vi "CollisionAvoidance.vi"(8 "error in":errorcluster) -> (0 "error out":errorcluster)   [LabVIEW 2009, in "Main.lvlib"]
doc: "Collision Avoidance algorithm. Check if there is an obstacle in front and aborts position control if any."
uses:
  Main.lvlib
  Drive.lvlib
  MainVariables.lvlib
  ImageProject/Camera.lvlib
  NetworkVarTarget.lvlib
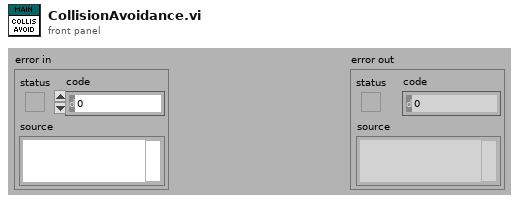
[diagram p1: front panel]
types:
  T1 = typedef "IMAQ Image.ctl" = refnum<image>
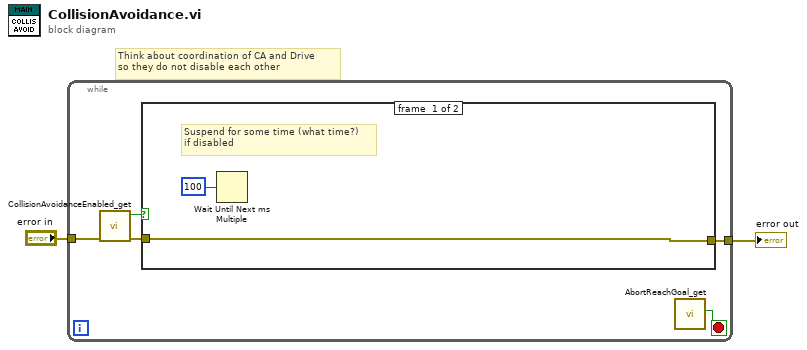
[diagram p0: block diagram]
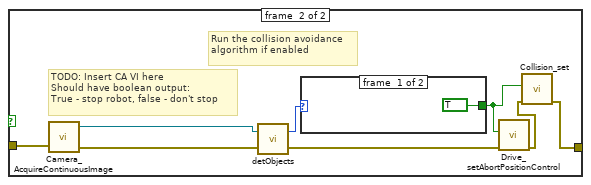
[diagram p2: hidden frame]
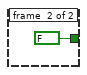
[diagram p3: hidden frame]
diagram:
  # "Think about coordination of CA and Drive\nso they do not disable each other"
  n1 = while {
    tunnel: [w5] -> w1
    tunnel: "error in" -> [w4]
    stop <- w3 stop-if-true
    n2 = call "CollisionAvoidanceEnabled_get.vi"("error in (no error)"=w4) -> ("error out"=w6:errorcluster, "Enabled"=w7:bool)  [unwired: 9 in]
    n3 = case shown="True" w7 {
      tunnel: w6 -> [w8 w15]
      tunnel: [w8 w11] -> w5
      frame #0 {
        # "Suspend for some time (what time?)\nif disabled"
        n4 = Wait Until Next ms Multiple(millisecond multiple=u32 100) -> ()  [unwired: 1 out]
      }
      frame #1 {
        # "Run the collision avoidance\nalgorithm if enabled"
        # "TODO: Insert CA VI here\nShould have boolean output:\nTrue - stop robot, false - don't stop"
        n5 = call "Camera_AcquireContinuousImage.vi"("error in"=w15) -> ("Image Out"=w17:T1, "error out"=w16:errorcluster)  [unwired: 1 in, 1 out]
        n6 = call "detObjects.vi"("error in (no error)"=w16, "Image in"=w17) -> ("error out"=w14:errorcluster, "Output"=w13:i32)
        n7 = case shown="0" w13 {
          tunnel: [TRUE ("Abort? (F)") FALSE ("Abort? (F)")] -> w10
          frame #0 {
          }
          frame #1 {
          }
        }
        n8 = call "Drive_setAbortPositionControl.vi"("error in (no error)"=w14, "Abort? (F)"=w10) -> ("error out"=w12:errorcluster)  [unwired: 9 in]
        n9 = call "Collision_set.vi"("error in (no error)"=w12, "Collision? (F)"=w10) -> ("error out"=w11:errorcluster)  [unwired: 9 in]
      }
    }
    n10 = call "AbortReachGoal_get.vi"() -> ("Abort"=w3:bool)  [unwired: 10 in, 1 out]
  }
  "error out" <- w1
